vi "Pre-Build Action - full.vi"(6 "Top Level/Always Included VIs":path[](array[path]), 7 "Main Destination Path":path, 9 "Target Name":string, 10 "Build Specification Name":string, 11 "Project Path":path) -> (0 "error out":errorcluster)   [LabVIEW 2020]
doc: "This vi is called by build as pre-build action. VI setup conditional symbols."
uses:
  <vilib>/Comparison/Equal/Equal Functor/Equal Functor.lvclass
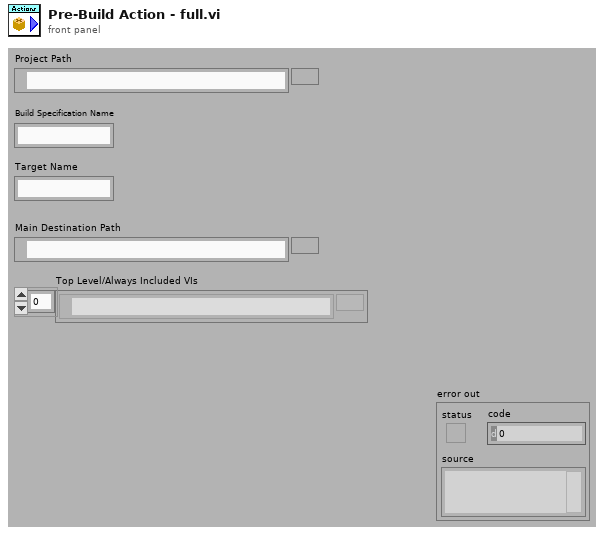
[diagram p1: front panel]
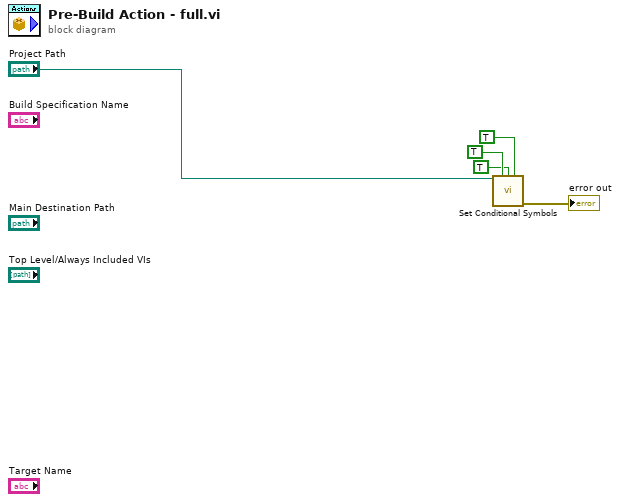
[diagram p0: block diagram]
diagram:
  n1 = call "Set Conditional Symbols.vi"("Project Path"="Project Path", "w_niscope"=TRUE, "w_visa"=TRUE, "w_daqmx"=TRUE) -> ("error out"=→"error out":errorcluster)  [unwired: 11 in]
